vi "señalizacion panel.vi"(3 "Mediciones M":T2, 4 "Config":T1, 5 "Eeprom D-cod":T5) -> (0 "POT=0":bool, 1 "Front leds":T3, 2 "Front meds":T4)   [LabVIEW 2010]
uses:
  <vilib>/Utility/error.llb/whitespace.ctl
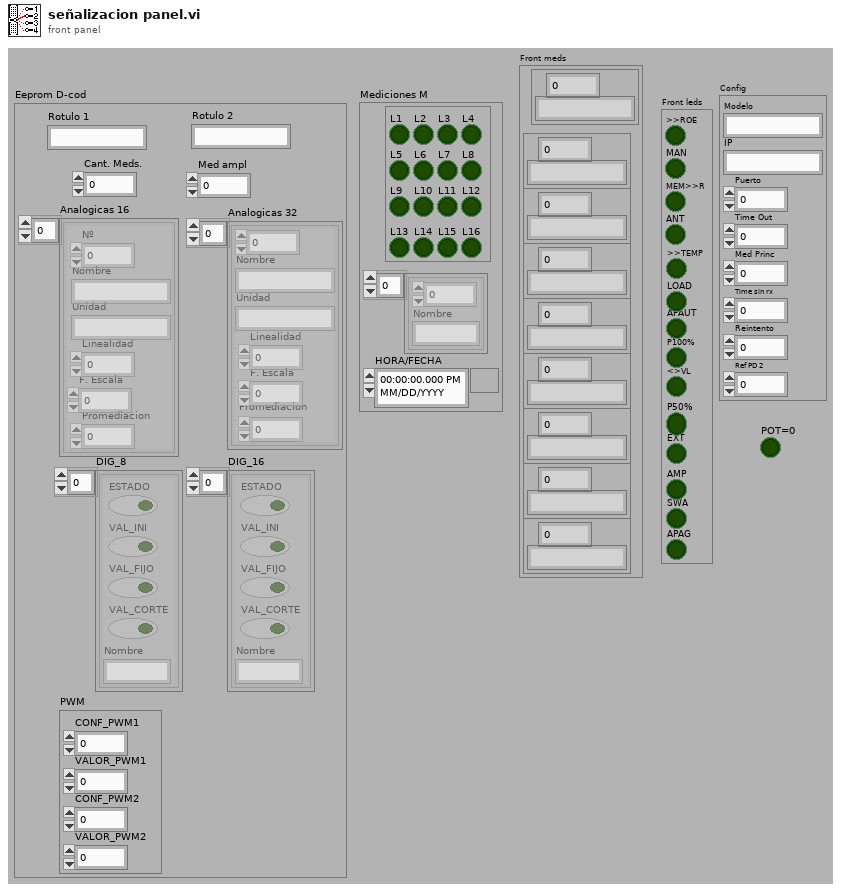
[diagram p1: front panel]
types:
  T1 = cluster{"Modelo":string, "IP":string, "Puerto":u16, "Time Out":u16, "Med Princ":u16, "Time sin rx":u16, "Reintento":u16, "Ref PD 2":u16}
  T2 = cluster{cluster{"L1":bool, "L2":bool, "L3":bool, "L4":bool, "L5":bool, "L6":bool, "L7":bool, "L8":bool, "L9":bool, "L10":bool, "L11":bool, "L12":bool, "L13":bool, "L14":bool, "L15":bool, "L16":bool}, cluster{dbl, "Nombre":string}[], "HORA/FECHA":timestamp}
  T3 = cluster{">>ROE":bool, "MAN":bool, "MEM>>R":bool, "ANT":bool, ">>TEMP":bool, "LOAD":bool, "APAUT":bool, "P100%":bool, "<>VL":bool, "P50%":bool, "EXT":bool, "AMP":bool, "SWA":bool, "APAG":bool}
  T4 = cluster{cluster{dbl, string}, cluster{dbl, string}, cluster{dbl, string}, cluster{dbl, string}, cluster{dbl, string}, cluster{dbl, string}, cluster{dbl, string}, cluster{dbl, string}, cluster{dbl, string}}
  T5 = cluster{"Rotulo 1":string, "Rotulo 2":string, "Cant. Meds.":u8, "Med ampl":u8, "Analogicas 16":cluster{"Nº":i32, "Nombre":string, "Unidad":string, "Linealidad":u8, "F. Escala":u8, "Promediacion":u8}[], "Analogicas 32":cluster{i32, "Nombre":string, "Unidad":string, "Linealidad":u8, "F. Escala":u8, "Promediacion":u8}[], "DIG_8":cluster{"ESTADO":bool, "VAL_INI":bool, "VAL_FIJO":bool, "VAL_CORTE":bool, "Nombre":string}[], "DIG_16":cluster{"ESTADO":bool, "VAL_INI":bool, "VAL_FIJO":bool, "VAL_CORTE":bool, "Nombre":string}[], "PWM":cluster{"CONF_PWM1":u8, "VALOR_PWM1":u8, "CONF_PWM2":u8, "VALOR_PWM2":u8}}
  T6 = typedef "whitespace.ctl" = u16
  T7 = cluster{"Nº":i32, "Nombre":string, "Unidad":string, "Linealidad":u8, "F. Escala":u8, "Promediacion":u8}[]
  T8 = cluster{i32, "Nombre":string, "Unidad":string, "Linealidad":u8, "F. Escala":u8, "Promediacion":u8}[]
  T9 = cluster{"Nº":i32, "Nombre":string, "Unidad":string, "Linealidad":u8, "F. Escala":u8, "Promediacion":u8}
  T10 = cluster{"L1":bool, "L2":bool, "L3":bool, "L4":bool, "L5":bool, "L6":bool, "L7":bool, "L8":bool, "L9":bool, "L10":bool, "L11":bool, "L12":bool, "L13":bool, "L14":bool, "L15":bool, "L16":bool}
  T11 = cluster{cluster{dbl, "trimmed string":string}, cluster{dbl, string}, cluster{dbl, string}, cluster{dbl, string}, cluster{dbl, string}, cluster{dbl, string}, cluster{dbl, string}, cluster{dbl, string}, cluster{dbl, string}}
  T12 = cluster{bool, bool, "L13":bool, bool, bool, "L15":bool, bool, bool, bool, bool, bool, bool, bool, bool}
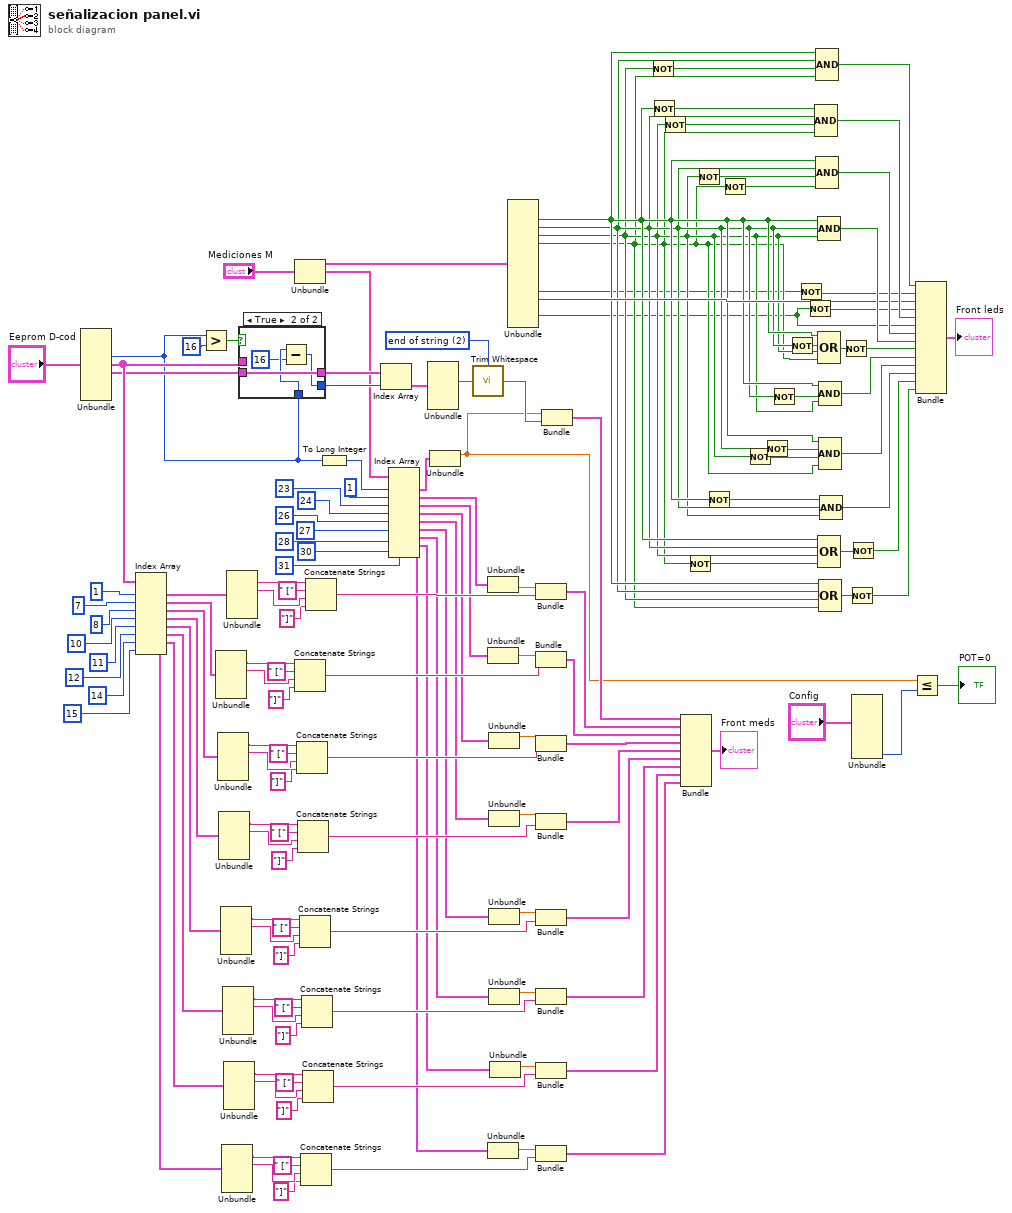
[diagram p0: block diagram]
diagram:
  w34 = T6 2 items=["both", "start of string", "end of string"] ("location (both)")
  n1 = Unbundle("Eeprom D-cod") -> ("Med ampl"=w39:u8, "Analogicas 16"=w144:T7, "Analogicas 32"=w94:T8)  [unwired: 6 out]
  n2 = Index Array(array=w144, index #1=1 ("index"), index #2=7 ("index"), index #3=8 ("index"), index #4=10 ("index"), index #5=11 ("index"), index #6=12 ("index"), index #7=14 ("index"), index #8=15 ("index")) -> (element #1=w143:T9, element #2=w26:T9, element #3=w25:T9, element #4=w24:T9, element #5=w23:T9, element #6=w22:T9, element #7=w21:T9, element #8=w20:T9)
  n3 = Greater?(x=w39, y=u8 16) -> (0:w137:bool)
  n4 = Unbundle(w26) -> ("Nombre"=w127:string, "Unidad"=w126:string)  [unwired: 4 out]
  n5 = Unbundle(w25) -> ("Nombre"=w97:string, "Unidad"=w96:string)  [unwired: 4 out]
  n6 = Unbundle(w24) -> ("Nombre"=w104:string, "Unidad"=w105:string)  [unwired: 4 out]
  n7 = Unbundle(w23) -> ("Nombre"=w107:string, "Unidad"=w106:string)  [unwired: 4 out]
  n8 = Unbundle(w20) -> ("Nombre"=w114:string, "Unidad"=w115:string)  [unwired: 4 out]
  n9 = Unbundle(w22) -> ("Nombre"=w124:string, "Unidad"=w125:string)  [unwired: 4 out]
  n10 = Unbundle(w21) -> ("Nombre"=w117:string, "Unidad"=w116:string)  [unwired: 4 out]
  n11 = Unbundle(w143) -> ("Nombre"=w142:string, "Unidad"=w133:string)  [unwired: 4 out]
  n12 = case shown="True" w137 {
    tunnel: w144 -> [w147 _]
    tunnel: w94 -> [_ w151]
    tunnel: [w147 w151] -> w138
    tunnel: w39 -> [w146 w149]
    tunnel: [w146 w150] -> w140
    frame False {
    }
    frame True {
      n13 = Subtract(x=w149, y=u8 16) -> (x-y=w150:u8)
    }
  }
  n14 = Unbundle("Mediciones M") -> (w85:T10, w95:cluster{dbl, "Nombre":string}[])  [unwired: 1 out]
  n15 = Concatenate Strings(w127, " [" ("string"), w126, "]" ("string")) -> (w130:string)
  n16 = Concatenate Strings(w97, " [" ("string"), w96, "]" ("string")) -> (w100:string)
  n17 = Concatenate Strings(w104, " [" ("string"), w105, "]" ("string")) -> (w101:string)
  n18 = Concatenate Strings(w107, " [" ("string"), w106, "]" ("string")) -> (w110:string)
  n19 = Concatenate Strings(w114, " [" ("string"), w115, "]" ("string")) -> (w111:string)
  n20 = Concatenate Strings(w124, " [" ("string"), w125, "]" ("string")) -> (w121:string)
  n21 = Concatenate Strings(w117, " [" ("string"), w116, "]" ("string")) -> (w120:string)
  n22 = Concatenate Strings(w142, " [" ("string"), w133, "]" ("string")) -> (w131:string)
  n23 = To Long Integer(number=w39) -> (32bit integer=w5:i32)
  n24 = Index Array(array=w138, index=w140) -> (element=w139:T9)
  n25 = Index Array(array=w95, index #1=w5, index #2=1 ("index"), index #3=23 ("index"), index #4=24 ("index"), index #5=26 ("index"), index #6=27 ("index"), index #7=28 ("index"), index #8=30 ("index"), index #9=31 ("index")) -> (element #1=w4:cluster{dbl, "Nombre":string}, element #2=w48:cluster{dbl, "Nombre":string}, element #3=w19:cluster{dbl, "Nombre":string}, element #4=w11:cluster{dbl, "Nombre":string}, element #5=w10:cluster{dbl, "Nombre":string}, element #6=w9:cluster{dbl, "Nombre":string}, element #7=w8:cluster{dbl, "Nombre":string}, element #8=w7:cluster{dbl, "Nombre":string}, element #9=w6:cluster{dbl, "Nombre":string})
  n26 = Unbundle(w139) -> ("Unidad"=w35:string)  [unwired: 5 out]
  n27 = Unbundle(w4) -> (w1:dbl)  [unwired: 1 out]
  n28 = call <vilib>:"Trim Whitespace.vi"("string"=w35, "location (both)"=w34) -> ("trimmed string"=w2:string)
  n29 = Unbundle(w48) -> (w47:dbl)  [unwired: 1 out]
  n30 = Unbundle(w19) -> (w46:dbl)  [unwired: 1 out]
  n31 = Unbundle(w6) -> (w42:dbl)  [unwired: 1 out]
  n32 = Unbundle(w11) -> (w45:dbl)  [unwired: 1 out]
  n33 = Unbundle(w10) -> (w44:dbl)  [unwired: 1 out]
  n34 = Unbundle(w9) -> (w43:dbl)  [unwired: 1 out]
  n35 = Unbundle(w8) -> (w40:dbl)  [unwired: 1 out]
  n36 = Unbundle(w7) -> (w41:dbl)  [unwired: 1 out]
  n37 = Unbundle(w85) -> ("L3"=w63:bool, "L4"=w62:bool, "L5"=w61:bool, "L6"=w60:bool, "L12"=w58:bool, "L13"=w64:bool, "L15"=w56:bool)  [unwired: 9 out]
  n38 = Bundle(w47, w131) -> (w93:cluster{dbl, string})  [unwired: 1 in]
  n39 = Bundle(w46, w130) -> (w92:cluster{dbl, string})  [unwired: 1 in]
  n40 = Bundle(w45, w100) -> (w91:cluster{dbl, string})  [unwired: 1 in]
  n41 = Bundle(w44, w101) -> (w90:cluster{dbl, string})  [unwired: 1 in]
  n42 = Bundle(w43, w110) -> (w89:cluster{dbl, string})  [unwired: 1 in]
  n43 = Bundle(w40, w121) -> (w88:cluster{dbl, string})  [unwired: 1 in]
  n44 = Bundle(w41, w120) -> (w87:cluster{dbl, string})  [unwired: 1 in]
  n45 = Bundle(w42, w111) -> (w86:cluster{dbl, string})  [unwired: 1 in]
  n46 = Bundle(w1, "trimmed string"=w2) -> (w3:cluster{dbl, "trimmed string":string})  [unwired: 1 in]
  n47 = Not(x=w61) -> (.not. x?=w80:bool)
  n48 = Not(x=w63) -> (.not. x?=w79:bool)
  n49 = Not(x=w61) -> (.not. x?=w78:bool)
  n50 = Bundle(w3, w93, w92, w91, w90, w89, w88, w87, w86) -> (→"Front meds":T11)  [unwired: 1 in]
  n51 = Not(x=w60) -> (.not. x?=w72:bool)
  n52 = Not(x=w61) -> (.not. x?=w76:bool)
  n53 = Not(x=w63) -> (.not. x?=w71:bool)
  n54 = Not(x=w60) -> (.not. x?=w77:bool)
  n55 = Not(x=w61) -> (.not. x?=w69:bool)
  n56 = Not(x=w62) -> (.not. x?=w70:bool)
  n57 = Not(x=w62) -> (.not. x?=w68:bool)
  n58 = Not(x=w62) -> (.not. x?=w67:bool)
  n59 = Not(x=w58) -> (.not. x?=w59:bool)
  n60 = Not(x=w56) -> (.not. x?=w57:bool)
  n61 = Compound Arithmetic op=AND(w79, w62, w78, w60) -> (w82:bool)
  n62 = Compound Arithmetic op=AND(w63, w62, w80, w60) -> (w83:bool)
  n63 = Compound Arithmetic op=AND(w63, w62, w76, w77) -> (w81:bool)
  n64 = Compound Arithmetic op=AND(w63, w62, w61) -> (w84:bool)
  n65 = Compound Arithmetic op=OR(w63, w67, w61, w60) -> (w50:bool)
  n66 = Compound Arithmetic op=OR(w63, w62, w61, w72) -> (w53:bool)
  n67 = Compound Arithmetic op=AND(w63, w68, w61) -> (w75:bool)
  n68 = Compound Arithmetic op=AND(w63, w70, w69, w60) -> (w74:bool)
  n69 = Compound Arithmetic op=OR(w63, w62, w61, w60) -> (w55:bool)
  n70 = Compound Arithmetic op=AND(w71, w62, w61) -> (w73:bool)
  n71 = Not(x=w50) -> (.not. x?=w51:bool)
  n72 = Not(x=w55) -> (.not. x?=w54:bool)
  n73 = Not(x=w53) -> (.not. x?=w52:bool)
  n74 = Unbundle("Config") -> ("Ref PD 2"=w36:u16)  [unwired: 7 out]
  n75 = Less Or Equal?(x=w1, y=w36) -> (x <= y?=→"POT=0":bool)
  n76 = Bundle(w83, w59, "L13"=w64, w57, w82, "L15"=w56, w81, w84, w51, w75, w74, w73, w52, w54) -> (→"Front leds":T12)  [unwired: 1 in]
